vi "FPGA Encode NEW .vi"(8 "Direction":bool, 9 "Down":bool, 10 "Rise":bool, 11 "ENC":i32) -> (3 "ENC+":i32)   [LabVIEW 2017]
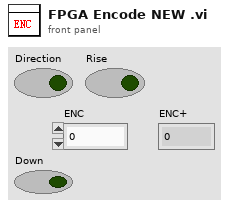
[diagram p1: front panel]
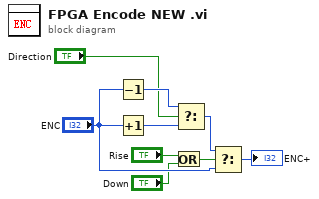
[diagram p0: block diagram]
diagram:
  n1 = Decrement(x="ENC") -> (x-1=w5:i32)
  n2 = Increment(x="ENC") -> (x+1=w6:i32)
  n3 = Or(x="Rise", y="Down") -> (x .or. y?=w2:bool)
  n4 = Select(t=w5, s="Direction", f=w6) -> (s? t:f=w7:i32)
  n5 = Select(t=w7, s=w2, f="ENC") -> (s? t:f=→"ENC+":i32)
